vi "Test Component A Does Yet Another Thing.vi"(11 "Test Case In":refnum<class "Component A Another Test.lvclass">) -> (0 "error out":errorcluster, 3 "Test Case Out":refnum<class "Component A Another Test.lvclass">)   [LabVIEW 2020, in "Component A Test Suite.lvlib" / "Component A Another Test.lvclass"]
uses:
  Component A Another Test.lvclass
  Component A Another Test.lvclass/Component A Another Test.ctl
  07093915-9c26-48f6-99f8-4375e800798e.vi
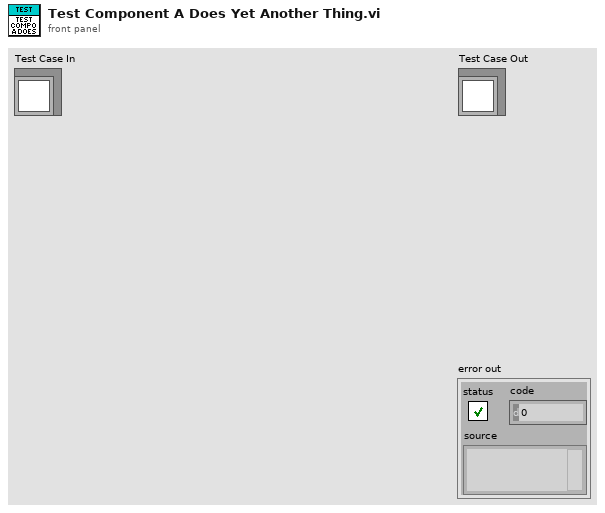
[diagram p1: front panel]
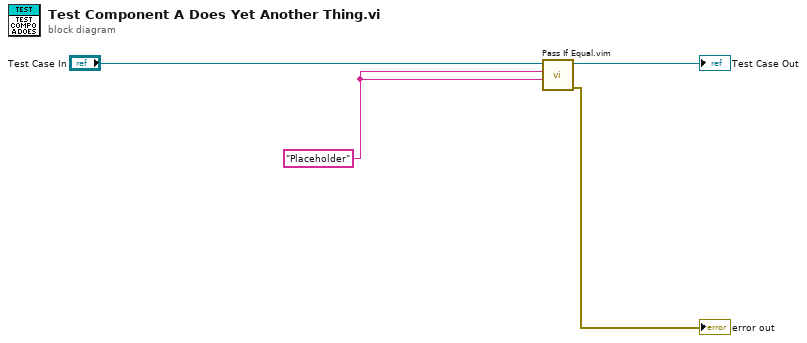
[diagram p0: block diagram]
diagram:
  w1 = "Placeholder"
  n1 = call "Pass If Equal.vim"("Actual"=w1, "Expected"=w1, "LUnit Test Case In"="Test Case In") -> ("error out"=→"error out":errorcluster, "LUnit Test Case Out"=→"Test Case Out":refnum<class "Component A Another Test.lvclass">)  [unwired: 7 in]
